vi "Global_An_In_Var.vi"() -> ()   [LabVIEW 2016, in "DNP3_Master_Station_Template.lvlib"]
uses:
  <vilib>/DNP3/DNP3_Master/Poll Analog Input Variation.ctl
  DNP3_Master_Station_Template.lvlib
  <vilib>/DNP3/DNP3_Master.lvlib
panel:
  in  "Analog In Variation":T1=6 items=["Default", "32-bit with Flag", "16-bit with Flag", "32-bit without Flag", "16-bit without Flag", "Single-prec with Flag", "Double-prec with Flag"]
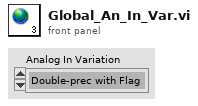
[diagram p1: front panel]
types:
  T1 = typedef "DNP3_Master.lvlib/Poll Analog Input Variation.ctl" = u8
diagram:
